vi "Theme4_Topic2_qn26.vi"(9 "RefPrevious":refnum<vi>, 10 "RefNext":refnum<vi>, 11 "connection reference":T1) -> (2 "AnsIndicator":refnum<vi>[](array[refnum]))   [LabVIEW 2013]
uses:
  why.vi
  Precontrol.vi
  <vilib>/addons/database/Connection.llb/Conn ObjectReference.ctl
  <vilib>/addons/database/NI_Database_API.lvlib
panel:
  out "Why?":string
  out "DInd":bool
  out "CInd":bool
  out "BInd":bool
  out "AInd":bool
  in  "ABCD":enum32{"No Selection", "A", "B", "C", "D"}(radio)
  out "MCQ_Randomized":string[](array[string])
  # "Given that the wave shown below has a frequency of 100 Hz . what is the speed of the wave ?"
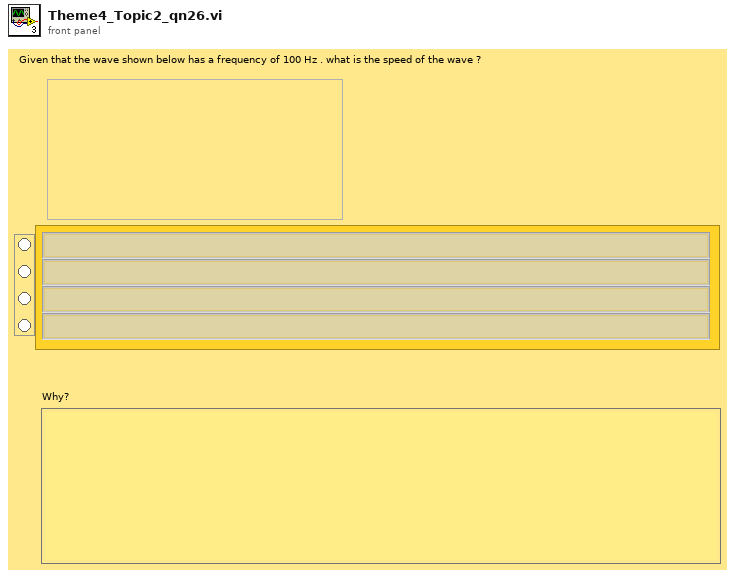
[diagram p1: front panel]
types:
  T1 = typedef "NI_Database_API.lvlib/Conn ObjectReference.ctl" = refnum<k1>
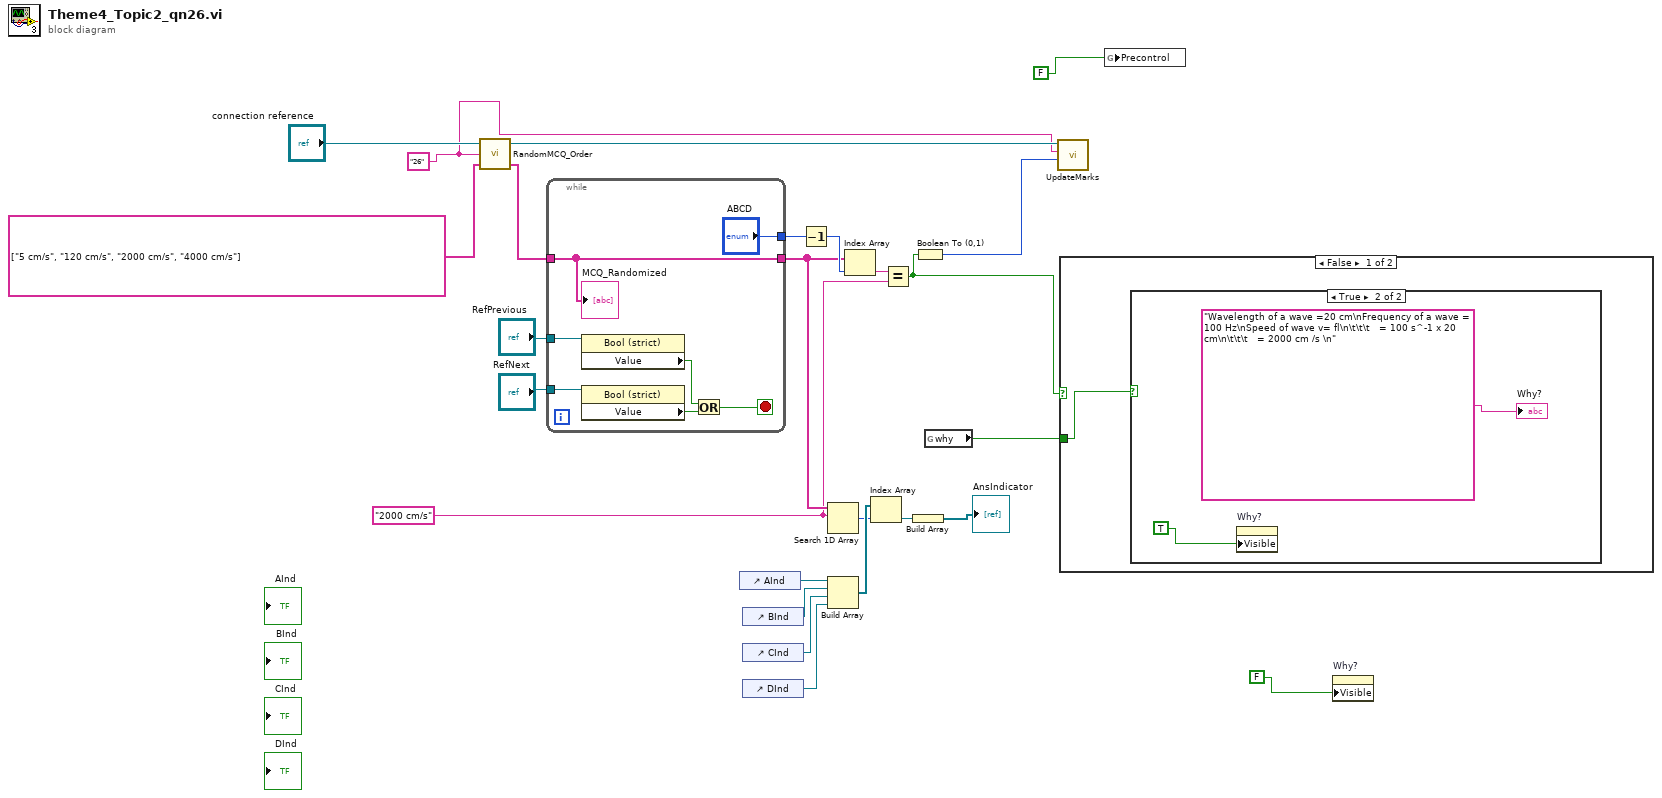
[diagram p0: block diagram]
diagram:
  w12 = "2000 cm/s" ("element")
  w3 = "26" ("Questions_Ordered")
  n1 = call "RandomMCQ_Order.vi"("MCQ_Ordered"=string[] ["5 cm/s", "120 cm/s", "2000 cm/s", "4000 cm/s"], "Questions_Ordered"=w3, "connection reference"="connection reference") -> ("MCQ_Randomized"=w25:string[], "connection reference out"=w10:T1)  [unwired: 1 in]
  n2 = while {
    tunnel: ["ABCD"] -> w2
    tunnel: w25 -> [w27]
    tunnel: [w27] -> w14
    tunnel: "RefNext" -> [w28]
    tunnel: "RefPrevious" -> [w29]
    stop <- w26 stop-if-true
    n3 = property class="Bool (strict)"(reference=w29) -> ("Value"=w31:bool)  [unwired: 1 in, 2 out]
    n4 = property class="Bool (strict)"(reference=w28) -> ("Value"=w30:bool)  [unwired: 1 in, 2 out]
    n5 = Or(x=w31, y=w30) -> (x .or. y?=w26:bool)
    "MCQ_Randomized" <- w27
  }
  n6 = control-ref of="AInd"() -> (w22:refnum<vi>)
  n7 = control-ref of="BInd"() -> (w21:refnum<vi>)
  n8 = control-ref of="CInd"() -> (w20:refnum<vi>)
  n9 = control-ref of="DInd"() -> (w19:refnum<vi>)
  n10 = Decrement(x=w2) -> (x-1=w15:enum32{"No Selection", "A", "B", "C", "D"})
  n11 = Search 1D Array(1D array=w14, element=w12) -> (index of element=w17:i32)  [unwired: 1 in]
  n12 = Build Array(w22, w21, w20, w19) -> (w18:refnum<vi>[])
  n13 = Index Array(array=w14, index=w15) -> (element=w13:string)
  n14 = Index Array(array=w18, index=w17) -> (element=w16:refnum<vi>)
  n15 = Equal?(x=w13, y=w12) -> (x = y?=w6:bool)
  n16 = Build Array(w16) -> (→"AnsIndicator":refnum<vi>[])
  n17 = Boolean To (0,1)(Boolean=w6) -> (0, 1=w7:i16)
  n18 = global read "why.vi" "why"() -> (w5:bool)
  n19 = call "UpdateMarks.vi"("MarksEarned"=w7, "QuestionsNo_Ordered"=w3, "connection reference"=w10) -> ()  [unwired: 9 in]
  n20 = case shown="False" w6 {
    tunnel: w5 -> [w33 _]
    frame False {
      n21 = case shown="True" w33 {
        frame False {
        }
        frame True {
          n22 = property on="Why?" class="Str"("Visible"=TRUE) -> ()  [unwired: 2 in, 2 out]
          "Why?" <- "Wavelength of a wave =20 cm\nFrequency of a wave = 100 Hz\nSpeed of wave v= fl\n\t\t\t   = 100 s^-1 x 20 cm\n\t\t\t   = 2000 cm /s \n"
        }
      }
    }
    frame True {
    }
  }
  n23 = global write "Precontrol.vi" "Precontrol"(FALSE) -> ()
  n24 = property on="Why?" class="Str"("Visible"=FALSE) -> ()  [unwired: 2 in, 2 out]
